vi "Programa VentMej.vi"() -> ()   [LabVIEW 2023]
uses:
  f4b1dcb5-f55f-46d8-b56b-cff1d6391f74.vi
  <vilib>/Utility/file.llb/Write Delimited Spreadsheet (DBL).vi
  <vilib>/Instr/_visa.llb/VISA Configure Serial Port (Instr).vi
panel:
  out "Irradiación\nterminada":bool
  out "Duración de la prueba":dbl format="%<%H:%M:%S>t"
  out "Porcentaje avance":u8(slide) scale=0.0..100.0
  out "Pulsos enviados":dbl
  in  "Ruta de archivo":path=path "C:/Users/arakh/Desktop/MejoraVI/CalibTeensy.txt"
  out "Serial Write":string="0,0,2450,1000,8,15,116\r\n"
  out "Serial Read":string="MicroMalaria, 0, 0, 2450, 1000, 8, 0, 0, 0\r\n"
  in  "Potencia de salida":i32=1000 min=10 max=60 step=1
  in  "Comenzar Irradiación":bool
  in  "Frecuencia de operación":i32=2450 min=0 max=1 step=1
  out "Fecha y Hora":timestamp=timestamp(3762046627.8618994 s since 1904-01-01) format="%<%X\n%x>T"
  in  "stop":bool
  in  "ON time (sec)":i32(slide)=8 scale=0.0..15.0
  in  "OFF time (sec)":i32(slide)=15 min=10 max=60 step=1 scale=0.0..20.0
  in  "Número de pulsos":i32(knob)=116 min=10 max=60 step=1 scale=0.0..200.0
  in  "Data storage":bool
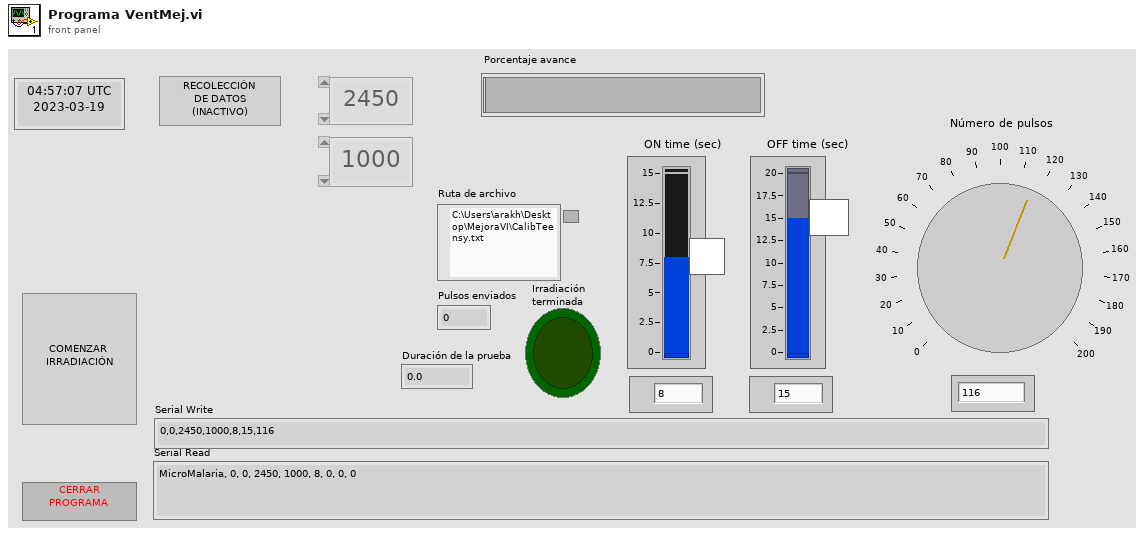
[diagram p1: front panel]
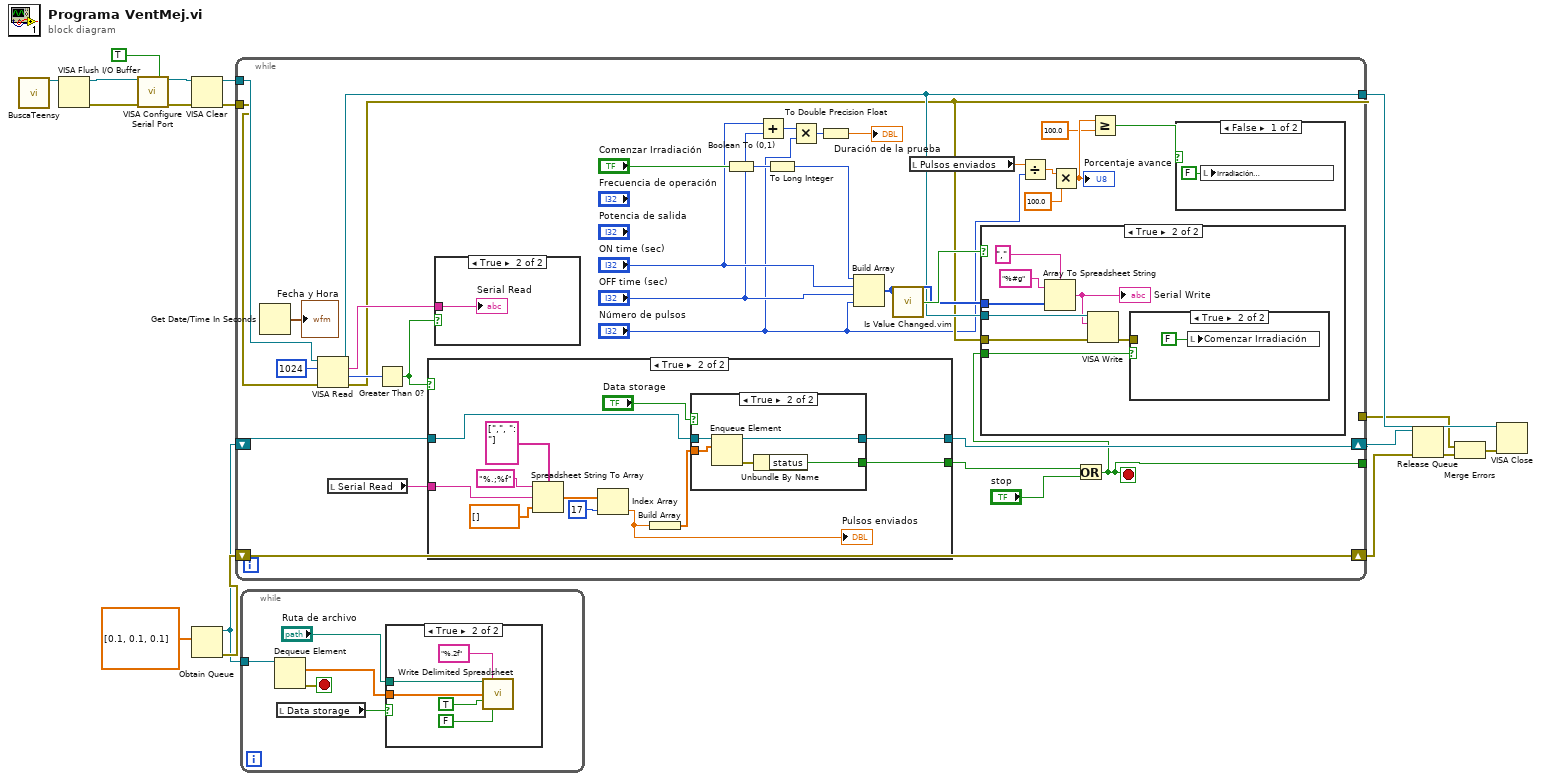
[diagram p0: block diagram]
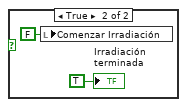
[diagram p3: hidden frame]
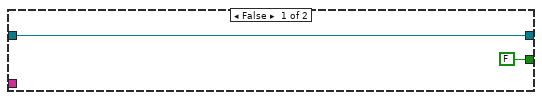
[diagram p4: hidden frame]
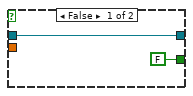
[diagram p5: hidden frame]
diagram:
  n1 = call "BuscaTeensy.vi"() -> ("VISA resource name out"=w9:refnum<visa-resource-name>)  [unwired: 15 in]
  n2 = VISA Flush I/O Buffer(VISA resource name=w9) -> (VISA resource name out=w11:refnum<visa-resource-name>, error out=w10:errorcluster)  [unwired: 2 in]
  n3 = call-poly "VISA Configure Serial Port"("VISA resource name"=w11, "Enable Termination\nChar (T)"=TRUE ("Enable Termination\nChar (T)"), "error in (no error)"=w10) -> ("VISA resource name out"=w15:refnum<visa-resource-name>, "error out"=w14:errorcluster)  [unwired: 11 in]
  n4 = VISA Clear(VISA resource name=w15, error in (no error)=w14) -> (VISA resource name out=w13:refnum<visa-resource-name>, error out=w12:errorcluster)
  n5 = Obtain Queue(element data type=dbl[] [0.1, 0.1, 0.1]) -> (queue out=w4:refnum<queue>, error out=w6:errorcluster)  [unwired: 4 in, 1 out]
  n6 = while {
    tunnel: [w34] -> w16
    tunnel: [w32] -> w2
    tunnel: w13 -> [w35]
    tunnel: w12 -> [w33]
    tunnel: [w38] -> _
    shift-right: [w37] -> w5
    shift-left: w6 -> [w37]
    shift-right: [w41] -> w7
    shift-left: w4 -> [w42]
    stop <- w38 stop-if-true
    n7 = Get Date/Time In Seconds() -> (seconds since 1Jan1904=→"Fecha y Hora":timestamp)
    n8 = VISA Read(VISA resource name=w35, byte count=u32 1024, error in (no error)=w33) -> (VISA resource name out=w34:refnum<visa-resource-name>, read buffer=w50:string, return count=w48:u32, error out=w32:errorcluster)
    n9 = local read "Serial Read"() -> (w31:string)
    n10 = Greater Than 0?(x=w48) -> (x > 0?=w30:bool)
    n11 = case shown="True" w30 {
      tunnel: w42 -> [w54 w59]
      tunnel: [w54 w58] -> w41
      tunnel: [FALSE ("status") w57] -> w39
      tunnel: w31 -> [_ w56]
      frame False {
      }
      frame True {
        n12 = Spreadsheet String To Array(delimiter (Tab)=string[] [",", ": "], format string="%.;%f", spreadsheet string=w56, array type (2D Dbl)=dbl[] []) -> (array=w64:dbl[])
        n13 = Index Array(array=w64, index=17) -> (element=w60:dbl)
        "Pulsos enviados" <- w60
        n14 = Build Array(w60) -> (w61:dbl[])
        n15 = case shown="True" "Data storage" {
          tunnel: w61 -> [_ w74]
          tunnel: w59 -> [w68 w73]
          tunnel: [w68 w72] -> w58
          tunnel: [FALSE ("status") w70] -> w57
          frame False {
          }
          frame True {
            n16 = Enqueue Element(queue=w73, element=w74) -> (queue out=w72:refnum<queue>, error out=w71:errorcluster)  [unwired: 2 in, 1 out]
            n17 = Unbundle By Name(w71) -> ("status"=w70:bool)
          }
        }
      }
    }
    n18 = case shown="True" w30 {
      tunnel: w50 -> [_ w75]
      frame False {
      }
      frame True {
        "Serial Read" <- w75
      }
    }
    n19 = Boolean To (0,1)(Boolean="Comenzar Irradiación") -> (0, 1=w43:i16)
    n20 = Add(x="ON time (sec)", y="OFF time (sec)") -> (x+y=w24:i32)
    n21 = To Long Integer(number=w43) -> (32bit integer=w36:i32)
    n22 = Multiply(x=w24, y="Número de pulsos") -> (x*y=w22:i32)
    n23 = To Double Precision Float(number=w22) -> (double precision float=→"Duración de la prueba":dbl)
    n24 = Build Array(w36, "ON time (sec)", "OFF time (sec)", "Número de pulsos") -> (w44:i32[])
    n25 = call "Is Value Changed.vim"("value"=w44) -> ("changed or first call?"=w47:bool)
    n26 = local read "Pulsos enviados"() -> (w29:dbl)
    n27 = Divide(x=w29, y="Número de pulsos") -> (x/y=w28:dbl)
    n28 = Multiply(x=w28, y=100.0) -> (x*y=w20:dbl)
    "Porcentaje avance" <- w20
    n29 = Or(x=w39, y="stop") -> (x .or. y?=w38:bool)
    n30 = case shown="True" w47 {
      tunnel: w34 -> [_ w81]
      tunnel: w32 -> [_ w80]
      tunnel: w44 -> [_ w79]
      tunnel: w38 -> [_ w77]
      frame False {
      }
      frame True {
        n31 = Array To Spreadsheet String(delimiter (Tab)=",", array=w79, 3:"%#g" ("format string")) -> (spreadsheet string=w76:string)
        "Serial Write" <- w76
        n32 = VISA Write(VISA resource name=w81, write buffer=w76, error in (no error)=w80) -> (error out=w78:errorcluster)  [unwired: 2 out]
        n33 = case shown="True" w77 {
          tunnel: w78 -> [_ _]
          frame False {
          }
          frame True {
            n34 = local write "Comenzar Irradiación"(FALSE ("Comenzar Respiración")) -> ()
          }
        }
      }
    }
    n35 = Greater Or Equal?(x=w20, y=100.0) -> (x >= y?=w18:bool)
    n36 = case shown="False" w18 {
      frame False {
        n37 = local write "Irradiación\nterminada"(FALSE ("Irradiación\nterminada")) -> ()
      }
      frame True {
        n38 = local write "Comenzar Irradiación"(FALSE ("Comenzar Irradiación")) -> ()
        "Irradiación\nterminada" <- TRUE ("Irradiación\nterminada")
      }
    }
  }
  n39 = while {
    tunnel: w4 -> [w86]
    stop <- w87 stop-if-true
    n40 = Dequeue Element(queue=w86) -> (element=w88:dbl[], error out=w87:errorcluster)  [unwired: 2 in, 2 out]
    n41 = local read "Data storage"() -> (w89:bool)
    n42 = case shown="True" w89 {
      tunnel: w88 -> [_ w91]
      tunnel: "Ruta de archivo" -> [_ w90]
      frame False {
      }
      frame True {
        n43 = call-poly <vilib>:"Write Delimited Spreadsheet.vi"("file path (dialog if empty)"=w90, "format (%.3f)"="%.2f", "1D data"=w91, "append to file? (new file:F)"=TRUE, "transpose? (no:F)"=FALSE) -> ()  [unwired: 9 in, 2 out]
      }
    }
  }
  n44 = Release Queue(queue=w7, error in (no error)=w5) -> (error out=w3:errorcluster)  [unwired: 1 in, 2 out]
  n45 = Merge Errors(w2, w3) -> (w1:errorcluster)
  n46 = VISA Close(VISA resource name=w16, error in (no error)=w1) -> ()  [unwired: 1 out]
